vi "Write MDA.vi"(8 "error in (no error)":errorcluster, 10 "MDA":T1, 11 "Airmar Data in":refnum<class "Airmar Data.lvclass">) -> (0 "error out":errorcluster, 3 "Airmar Data out":refnum<class "Airmar Data.lvclass">)   [LabVIEW 2013, in "Airmar Data.lvclass"]
uses:
  Airmar Data.lvclass
  Airmar Data.lvclass/Airmar Data.ctl
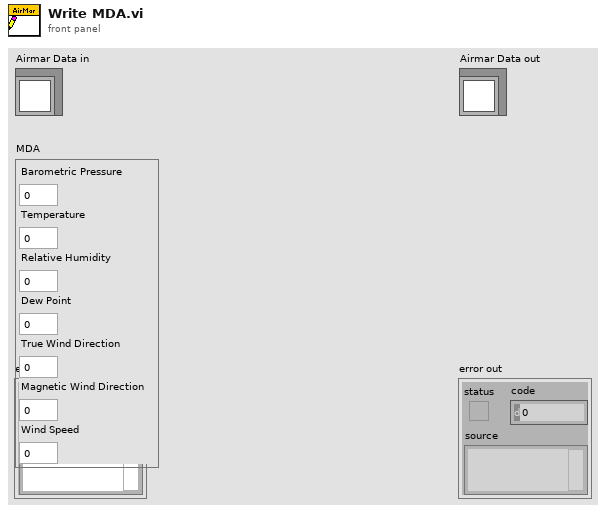
[diagram p1: front panel]
types:
  T1 = cluster{"Barometric Pressure":dbl, "Temperature":dbl, "Relative Humidity":dbl, "Dew Point":dbl, "True Wind Direction":dbl, "Magnetic Wind Direction":dbl, "Wind Speed":dbl}
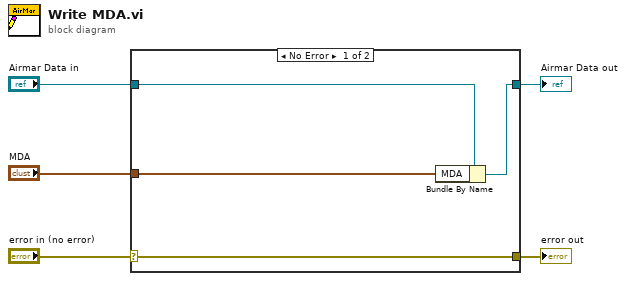
[diagram p0: block diagram]
diagram:
  n1 = case shown="No Error" "error in (no error)" {
    selector: "error in (no error)" -> [w9 w10]
    tunnel: [w9 w10] -> w4
    tunnel: [w7 w11] -> w2
    tunnel: "Airmar Data in" -> [w8 w11]
    tunnel: "MDA" -> [w6 _]
    frame No Error {
      n2 = Bundle By Name(cluster=w8, "MDA"=w6) -> (w7:refnum<class "Airmar Data.lvclass">)
    }
    frame Error {
    }
  }
  "error out" <- w4
  "Airmar Data out" <- w2
